vi "Stop Core.vi"(10 "final error code":i32, 11 "Measurement in":refnum<class "Measurement.lvclass">) -> (3 "Measurement out":refnum<class "Measurement.lvclass">)   [LabVIEW 2020, in "Measurement.lvlib" / "Measurement.lvclass"]
doc: "(<B>Filename</B>: Actor Framework.lvlib:Actor.lvclass:Stop Core.vi)\n\nDefines what the actor does before it stops. Use the <B>final error code</B> input to determine whether the actor shut down in response to an error.\n\nBy default, this method passes the Stop message along to all auto-stop nested actors. A descendant class may override this method to define additional behavior, such as shutting down any processes the actor initiated in its override of the Actor Core method."
uses:
  Measurement.lvclass
  <vilib>/ActorFramework/Actor/Actor.lvclass
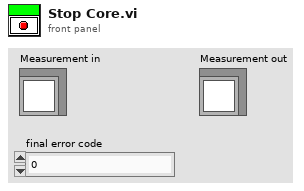
[diagram p1: front panel]
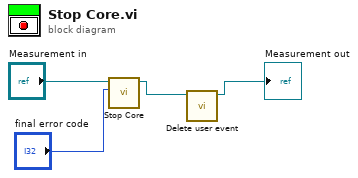
[diagram p0: block diagram]
diagram:
  n1 = call-parent "Stop Core.vi"("final error code"="final error code", "Actor in"="Measurement in") -> ("Actor out"=w2:refnum<class "Measurement.lvclass">)  [unwired: 9 in]
  n2 = call "Delete user event.vi"("Measurement in"=w2) -> ("Measurement out"=→"Measurement out":refnum<class "Measurement.lvclass">)  [unwired: 9 in, 1 out]
